vi "Create PUBLISH Packet (Client).vi"(4 "RETAIN":bool, 5 "PUBLISH type":refnum<class "PUBLISH.lvclass">, 6 "QoS":T1, 7 "DUP (Re-delivery attempt)":bool, 8 "error in (no error)":errorcluster, 9 "Packet ID (empty: generate new)":u16 format="%04x", 10 "Payload":u8[](array[numeric]) format="%08b", 11 "Topic Name":string) -> (0 "error out":errorcluster, 1 "Packet ID":u16 format="%04x", 3 "PUBLISH":refnum<class "PUBLISH.lvclass">)   [LabVIEW 2013, in "PUBLISH.lvclass"]
uses:
  PUBLISH.lvclass
  ControlPacket/QualityOfService -- enum.ctl
  ControlPacket/ControlPacket.lvclass/ControlPacket.ctl
  ControlPacket/ControlPacket.lvclass
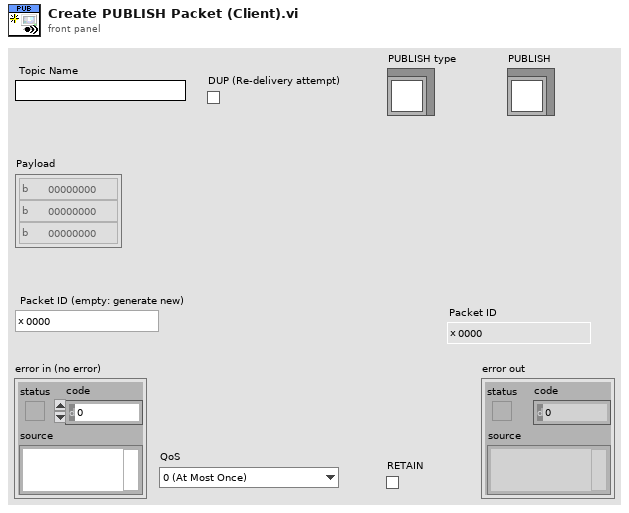
[diagram p1: front panel]
types:
  T1 = typedef "ControlPacket.lvclass/QualityOfService -- enum.ctl" = enum16{"0 (At Most Once)", "1 (At Least Once)", "2 (Exactly Once)"}
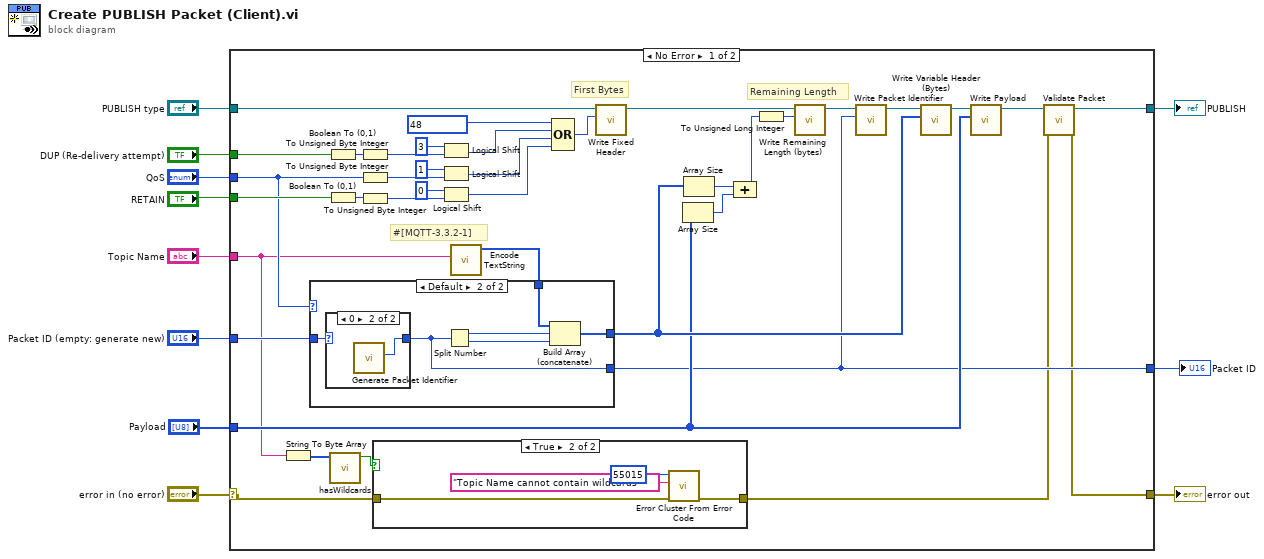
[diagram p0: block diagram]
diagram:
  n1 = case shown="No Error" "error in (no error)" {
    selector: "error in (no error)" -> [w13 w65]
    tunnel: [w18 w65] -> w10
    tunnel: [w19 w64] -> w8
    tunnel: "PUBLISH type" -> [w35 w64]
    tunnel: "DUP (Re-delivery attempt)" -> [w36 _]
    tunnel: "RETAIN" -> [w49 _]
    tunnel: "QoS" -> [w17 _]
    tunnel: "Topic Name" -> [w15 _]
    tunnel: "Packet ID (empty: generate new)" -> [w22 _]
    tunnel: "Payload" -> [w28 _]
    tunnel: [w21 _] -> w1
    frame No Error {
      # "#[MQTT-3.3.2-1]"
      # "Remaining Length"
      # "First Bytes"
      n2 = String To Byte Array(string=w15) -> (unsigned byte array=w16:u8[])
      n3 = Boolean To (0,1)(Boolean=w36) -> (0, 1=w45:i16)
      n4 = Boolean To (0,1)(Boolean=w49) -> (0, 1=w44:i16)
      n5 = call "hasWildcards.vi"("Topic Name (Bytes Array)"=w16) -> ("has Wildcards"=w14:bool)  [unwired: 10 in]
      n6 = To Unsigned Byte Integer(number=w45) -> (unsigned 8bit integer=w46:u8)
      n7 = To Unsigned Byte Integer(number=w17) -> (unsigned 8bit integer=w43:u8)
      n8 = To Unsigned Byte Integer(number=w44) -> (unsigned 8bit integer=w42:u8)
      n9 = case shown="True" w14 {
        tunnel: w13 -> [w50 w53]
        tunnel: [w50 w54] -> w12
        frame False {
        }
        frame True {
          n10 = call <vilib>:"Error Cluster From Error Code.vi"("error in (no error)"=w53, "error message (\"\")"="Topic Name cannot contain wildcards" ("error message (\"\")"), "error code (0)"=55015) -> ("error out"=w54:errorcluster)  [unwired: 6 in]
        }
      }
      n11 = Logical Shift(y=i16 3, x=w46) -> (x << y=w47:u8)
      n12 = Logical Shift(y=i16 1, x=w43) -> (x << y=w41:u8)
      n13 = Logical Shift(y=i16 0, x=w42) -> (x << y=w40:u8)
      n14 = call "Encode TextString.vi"("Text String"=w15) -> ("Length-Prefixed Field"=w30:u8[])  [unwired: 10 in]
      n15 = case shown="Default" w17 {
        tunnel: w30 -> [w55 w61]
        tunnel: [w55 w58] -> w29
        tunnel: w22 -> [_ w57]
        tunnel: [_ w56] -> w21
        frame "0 (At Most Once)" {
          # "#[MQTT-2.3.1-5]"
        }
        frame Default {
          n16 = case shown="0" w57 {
            selector: w57 -> [w62 _]
            tunnel: [w62 w63] -> w56
            frame Default {
            }
            frame 0 {
              n17 = call "Generate Packet Identifier.vi"() -> ("Packet Identifier"=w63:u16)  [unwired: 11 in]
            }
          }
          n18 = Split Number(x=w56) -> (hi(x)=w60:u8, lo(x)=w59:u8)
          n19 = Build Array (concatenate)(w61, w60, w59) -> (w58:u8[])
        }
      }
      n20 = Compound Arithmetic op=OR(u8 48, w47, w41, w40) -> (w34:u8)
      n21 = call "Write Fixed Header.vi"("Fixed Header"=w34, "ControlPacket in"=w35) -> ("ControlPacket out"=w32:refnum<class "PUBLISH.lvclass">)  [unwired: 9 in]
      n22 = Array Size(array=w28) -> (size(s)=w26:i32)
      n23 = Array Size(array=w29) -> (size(s)=w27:i32)
      n24 = Compound Arithmetic op=ADD(w27, w26) -> (w25:i32)
      n25 = To Unsigned Long Integer(number=w25) -> (unsigned 32bit integer=w33:u32)
      n26 = call "Write Remaining Length (bytes).vi"("Remaining Length (bytes)"=w33, "ControlPacket in"=w32) -> ("ControlPacket out"=w24:refnum<class "PUBLISH.lvclass">)  [unwired: 9 in]
      n27 = call "Write Packet Identifier.vi"("Packet Identifier"=w21, "ControlPacket in"=w24) -> ("ControlPacket out"=w23:refnum<class "PUBLISH.lvclass">)  [unwired: 9 in]
      n28 = call "Write Variable Header (Bytes).vi"("Variable Header (Bytes)"=w29, "ControlPacket in"=w23) -> ("ControlPacket out"=w31:refnum<class "PUBLISH.lvclass">)  [unwired: 9 in]
      n29 = call "Write Payload.vi"("Payload"=w28, "ControlPacket in"=w31) -> ("ControlPacket out"=w20:refnum<class "PUBLISH.lvclass">)  [unwired: 9 in]
      n30 = call "Validate Packet.vi"("error in (no error)"=w12, "ControlPacket in"=w20) -> ("error out"=w18:errorcluster, "ControlPacket out"=w19:refnum<class "PUBLISH.lvclass">)  [unwired: 8 in]
    }
    frame Error {
    }
  }
  "error out" <- w10
  "PUBLISH" <- w8
  "Packet ID" <- w1
